vi "[GV]_SPEED0.vi"() -> ()   [LabVIEW 2016]
panel:
  in  "SPEED0":u16
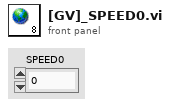
[diagram p1: front panel]
diagram:
